vi "TCP schreiben - FTIR.vi"(8 "error in":errorcluster caption="error out", 9 "Timeout schreiben":i32=190, 10 "String":string, 11 "connection ID":refnum<k5>) -> (0 "error out":errorcluster, 2 "Verknüpfter String":string, 3 "connection ID":refnum<k5>)   [LabVIEW 2020, in "FT-IR.lvlib" / "AK-Interface.lvlib"]
uses:
  AK-Interface.lvlib
panel:
  # "Ablaufinvariante Ausführung"
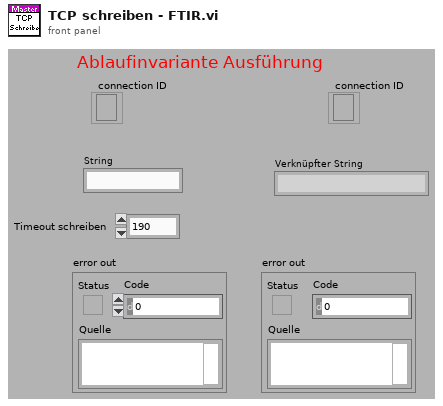
[diagram p1: front panel]
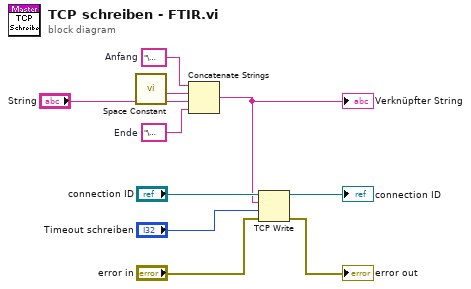
[diagram p0: block diagram]
diagram:
  w3 = "\u0002"  # Anfang
  w6 = "\u0003"  # Ende
  n1 = call <vilib>:"Space Constant.vi"() -> ("String"=w2:string)
  n2 = Concatenate Strings(w3, w2, "String", w6) -> (w4:string)
  "Verknüpfter String" <- w4
  n3 = TCP Write(connection ID="connection ID", data in=w4, error in (no error)="error in", 9:"Timeout schreiben") -> (connection ID out=→"connection ID":refnum<k5>, error out=→"error out":errorcluster)  [unwired: 1 out]
